vi "Read CAN Frames.vi"(8 "error in (no error)":errorcluster, 9 "Timeout (ms)":i32, 11 "Rx FIFO":refnum<k33>) -> (0 "error out":errorcluster, 2 "Frames":T1[](array[typedef]) {"payload" format="%x"; "timestamp" format="%<%.7X\n%x>T"; "type" items=["CAN Data"=0, "CAN Remote"=1, "CAN Bus Error"=2, "CAN 2.0 Data"=8, "CAN FD Data"=16, "CAN FD+BRS Data"=24, "J1939 Data"=192, "Delay"=224, "Log Trigger"=225, "Start Trigger"=226]; "identifier" format="%x"})   [LabVIEW 2020, in "985x Support Addon Engine.lvlib"]
uses:
  985x Support Addon Engine.lvlib
  <vilib>/xnet/xnet.llb/XNET Frame CAN.ctl
  <vilib>/xnet/xnet.llb/XNET Frame Type CAN.ctl
  <vilib>/xnet/xnet.llb/_XNET Convert Time U64 to LV.vi
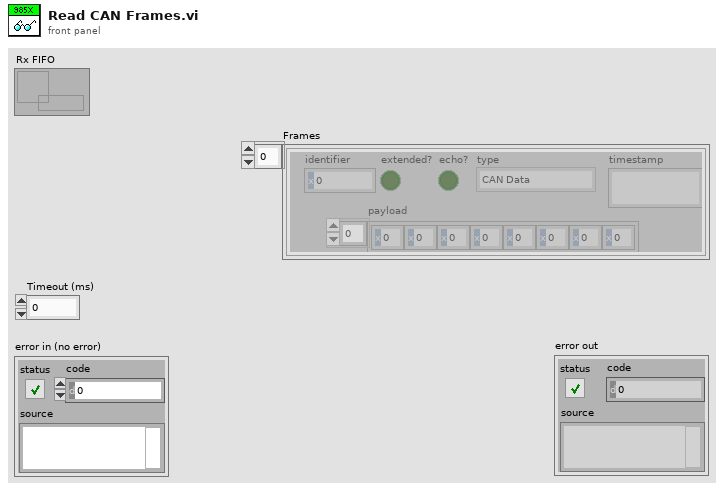
[diagram p1: front panel]
types:
  T1 = typedef "XNET Frame CAN.ctl" = cluster{"timestamp":timestamp, "payload":u8[], "identifier":u32, "type":T2, "extended?":bool, "echo?":bool}
  T2 = typedef "XNET Frame Type CAN.ctl" = u8
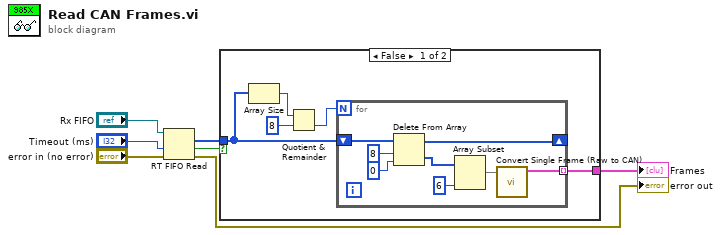
[diagram p0: block diagram]
diagram:
  n1 = RT FIFO Read(0:"Rx FIFO", 2:"Timeout (ms)", 3:"error in (no error)") -> (9:w3:u32[], 10:w4:bool, 11:→"error out":errorcluster)  [unwired: 1 in, 2 out]
  n2 = case shown="False" w4 {
    tunnel: w3 -> [w11 _]
    tunnel: [w12 _] -> w2
    frame False {
      n3 = Array Size(array=w11) -> (size(s)=w10:i32)
      n4 = Quotient & Remainder(x=w10, y=8) -> (floor(x/y)=w8:i32)  [unwired: 1 out]
      n5 = for {
        N: w8 -> [_]
        tunnel: [w20] -> w12 mode=indexing
        shift-right: [w18] -> _
        shift-left: w11 -> [w19]
        n6 = Delete From Array(array=w19, length=8, index=0 ("length")) -> (deleted portion=w15:u32[], array with subset deleted=w18:u32[])
        n7 = Array Subset(array=w15, length=6) -> (w14:u32[])  [unwired: 1 in]
        n8 = call "Convert Single Frame (Raw to CAN).vi"("Raw U32"=w14) -> ("CAN frame"=w20:T1)  [unwired: 8 in, 1 out]
      }
    }
    frame True {
    }
  }
  "Frames" <- w2
